vi "setLaserState.vi"(4 "error in (no error)":errorcluster, 7 "New Laser Status":bool) -> (0 "error out":errorcluster)   [LabVIEW 2024]
uses:
  OVA32.dll
panel:
  out "DLL Return Code":i32
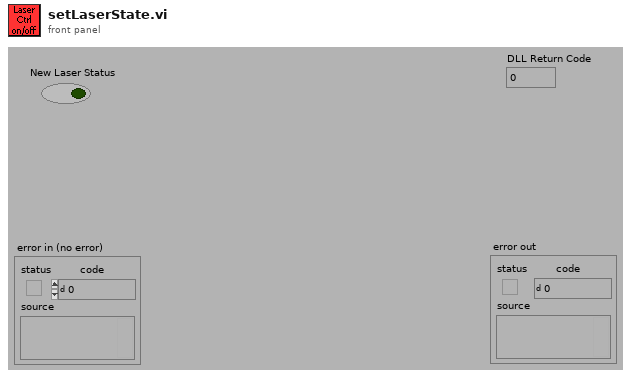
[diagram p1: front panel]
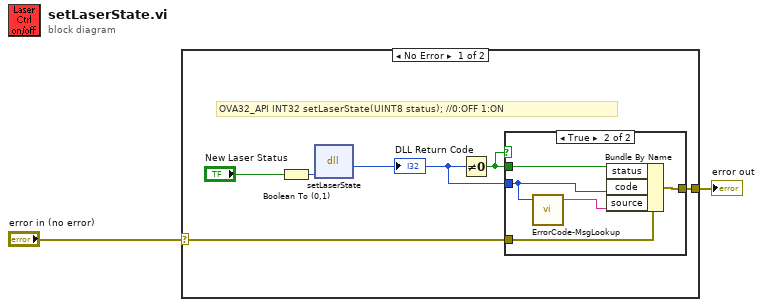
[diagram p0: block diagram]
diagram:
  n1 = case shown="No Error" "error in (no error)" {
    selector: "error in (no error)" -> [w3 w15]
    tunnel: [w8 w15] -> w2
    frame No Error {
      # "OVA32_API INT32 setLaserState(UINT8 status); //0:OFF 1:ON"
      n2 = Boolean To (0,1)(Boolean="New Laser Status") -> (0, 1=w6:i16)
      n3 = dll-call lib="OVA32.dll" fn="setLaserState"("status"=w6) -> (w7:i32)  [unwired: 4 in, 2 out]
      "DLL Return Code" <- w7
      n4 = Not Equal To 0?(x=w7) -> (x != 0?=w4:bool)
      n5 = case shown="True" w4 {
        tunnel: w3 -> [w9 w14]
        tunnel: w4 -> [_ w13]
        tunnel: [w9 w12] -> w8
        tunnel: w7 -> [_ w11]
        frame False {
        }
        frame True {
          n6 = call "ErrorCode-MsgLookup.vi"("DLL Return Code"=w11) -> ("Error String"=w10:string)  [unwired: 2 in, 2 out]
          n7 = Bundle By Name(cluster=w14, "status"=w13, "code"=w11, "source"=w10) -> (w12:errorcluster)
        }
      }
    }
    frame Error {
    }
  }
  "error out" <- w2
